vi "(SubVI)Waveform Editor_Import Manager_TextFile.vi"(6 "WF List_Sampling Rate":u32, 7 "New?":bool=TRUE, 8 "error in (no error)":errorcluster caption="에러 입력(에러 없음)", 10 "File Path":path=path "C:/Users/Oh Dae Woong/Desktop/test 221228.txt", 11 "Text File.lvclass":refnum<class "Text File.lvclass">) -> (0 "error out":errorcluster caption="에러 출력", 2 "Apply?":bool, 3 "Text File 출력":refnum<class "Text File.lvclass">)   [LabVIEW 2020]
uses:
  Libraries/Waveform Obj Class/Text File/Text File.lvclass
  Libraries/Waveform Obj Class/Waveform Obj/Waveform Obj.lvclass
  Libraries/Haptic IC Class/Haptic IC/Controls/(Ctrl)IC Type.ctl
  <vilib>/Utility/miscctls.llb/LVPointTypeDef.ctl
  Libraries/Waveform Obj Class/Waveform Obj/Waveform Obj.lvclass/Waveform Obj.ctl
  Libraries/Waveform Obj Class/Text File/Text File.lvclass/Text File.ctl
  Libraries/Waveform Obj Class/PWL_DW7802/PWL_DW7802.lvclass
  Libraries/Waveform Obj Class/PWL/PWL.lvclass/PWL.ctl
  Libraries/Waveform Obj Class/Waveform Gen/Waveform Gen.lvclass/Waveform Gen.ctl
  Libraries/Waveform Obj Class/Waveform Obj/Accessors/Read name.vi
  Libraries/Waveform Obj Class/Text File/Accessors/Read Text_Format.vi
  Libraries/Waveform Obj Class/Text File/Accessors/Read Text_Data.vi
  Libraries/Waveform Obj Class/Text File/Accessors/Read voltage idx.vi
  Libraries/Waveform Obj Class/Waveform Obj/Accessors/Read wait.vi
  Libraries/Waveform Obj Class/Waveform Obj/Accessors/Write sampling rate.vi
  Libraries/Waveform Obj Class/Text File/Accessors/Read Text_Sampling Rate.vi
  Libraries/Waveform Obj Class/Text File/Accessors/Read Text_ic type.vi
  Libraries/Waveform Obj Class/Waveform Obj/Accessors/Read play mode.vi
  Libraries/Waveform Obj Class/Text File/Accessors/Read Data.vi
  Libraries/Waveform Obj Class/Waveform Obj/Accessors/Write name.vi
  Libraries/Waveform Obj Class/PWL/Accessors/Write waveform type.vi
  Libraries/Waveform Obj Class/Waveform Gen/Accessors/Write repeat type.vi
  Libraries/Waveform Obj Class/Waveform Gen/Accessors/Write scale.vi
  Libraries/Waveform Obj Class/Waveform Gen/Accessors/Write frequency.vi
  Libraries/Waveform Obj Class/Waveform Gen/Accessors/Write cycle.vi
  Libraries/Waveform Obj Class/Waveform Obj/Accessors/Write play mode.vi
  Libraries/Waveform Obj Class/Waveform Obj/Accessors/Write voltage range.vi
  Libraries/Waveform Obj Class/PWL/Accessors/Write previous pwl scale.vi
  Libraries/Waveform Obj Class/Text File/Accessors/Read Text_File_PWL.vi
  Libraries/Waveform Obj Class/Waveform Obj/Accessors/Read sampling rate.vi
  Libraries/Waveform Obj Class/Text File/Accessors/Write voltage idx.vi
  Libraries/Waveform Obj Class/Waveform Obj/Accessors/Write wait.vi
  Libraries/Waveform Obj Class/Text File/Accessors/Read Error_.vi
  Libraries/Waveform Obj Class/Text File/Accessors/Read Memory Set.vi
  Variables/(Var)System Variables.vi
  <vilib>/Utility/file.llb/Write Delimited Spreadsheet (string).vi
  Libraries/Haptic IC Class/Haptic IC/Haptic IC.lvclass
panel:
  out "WAV_Sampling Rate":u32 caption="Sampling Rate" format="%#pHz"
  in  "Voltage Range":dbl(ring) caption="VD Clamp" items=["0.00V"=0.0, "0.04V"=0.04, "0.08V"=0.08, "0.12V"=0.12, "0.16V"=0.16, "0.20V"=0.2, "0.24V"=0.24, "0.28V"=0.28, "0.32V"=0.32, "0.36V"=0.36, "0.40V"=0.4, "0.44V"=0.44, "0.48V"=0.48, "0.52V"=0.52, "0.56V"=0.56, "0.60V"=0.6, "0.64V"=0.64, "0.68V"=0.68, "0.72V"=0.72, "0.76V"=0.76, "0.80V"=0.8, "0.84V"=0.84, "0.88V"=0.88, "0.92V"=0.92, "0.96V"=0.96, "1.00V"=1.0, "1.04V"=1.04, "1.08V"=1.08, "1.12V"=1.12, "1.16V"=1.16, "1.20V"=1.2, "1.24V"=1.24, "1.28V"=1.28, "1.32V"=1.32, "1.36V"=1.36, "1.40V"=1.4, "1.44V"=1.44, "1.48V"=1.48, "1.52V"=1.52, "1.56V"=1.56, "1.60V"=1.6, "1.64V"=1.64, "1.68V"=1.68, "1.72V"=1.72, "1.76V"=1.76, "1.80V"=1.8, "1.84V"=1.84, "1.88V"=1.88, "1.92V"=1.92, "1.96V"=1.96, "2.00V"=2.0, "2.04V"=2.04, "2.08V"=2.08, "2.12V"=2.12, "2.16V"=2.16, "2.20V"=2.2, "2.24V"=2.24, "2.28V"=2.28, "2.32V"=2.32, "2.36V"=2.36, "2.40V"=2.4, "2.44V"=2.44, "2.48V"=2.48, "2.52V"=2.52, "2.56V"=2.56, "2.60V"=2.6, "2.64V"=2.64, "2.68V"=2.68, "2.72V"=2.72, "2.76V"=2.76, "2.80V"=2.8, "2.84V"=2.84, "2.88V"=2.88, "2.92V"=2.92, "2.96V"=2.96, "3.00V"=3.0, "3.04V"=3.04, "3.08V"=3.08, "3.12V"=3.12, "3.16V"=3.16, "3.20V"=3.2, "3.24V"=3.24, "3.28V"=3.28, "3.32V"=3.32, "3.36V"=3.36, "3.40V"=3.4, "3.44V"=3.44, "3.48V"=3.48, "3.52V"=3.52, "3.56V"=3.56, "3.60V"=3.6, "3.64V"=3.64, "3.68V"=3.68, "3.72V"=3.72, "3.76V"=3.76, "3.80V"=3.8, "3.84V"=3.84, "3.88V"=3.88, "3.92V"=3.92, "3.96V"=3.96, "4.00V"=4.0, "4.04V"=4.04, "4.08V"=4.08, "4.12V"=4.12, "4.16V"=4.16, "4.20V"=4.2, "4.24V"=4.24, "4.28V"=4.28, "4.32V"=4.32, "4.36V"=4.36, "4.40V"=4.4, "4.44V"=4.44, "4.48V"=4.48, "4.52V"=4.52, "4.56V"=4.56, "4.60V"=4.6, "4.64V"=4.64, "4.68V"=4.68, "4.72V"=4.72, "4.76V"=4.76, "4.80V"=4.8, "4.84V"=4.84, "4.88V"=4.88, "4.92V"=4.92, "4.96V"=4.96, "5.00V"=5.0, "5.04V"=5.04, "5.08V"=5.08, "5.12V"=5.12, "5.16V"=5.16, "5.20V"=5.2, "5.24V"=5.24, "5.28V"=5.28, "5.32V"=5.32, "5.36V"=5.36, "5.40V"=5.4, "5.44V"=5.44, "5.48V"=5.48, "5.52V"=5.52, "5.56V"=5.56, "5.60V"=5.6, "5.64V"=5.64, "5.68V"=5.68, "5.72V"=5.72, "5.76V"=5.76, "5.80V"=5.8, "5.84V"=5.84, "5.88V"=5.88, "5.92V"=5.92, "5.96V"=5.96, "6.00V"=6.0, "6.04V"=6.04, "6.08V"=6.08, "6.12V"=6.12, "6.16V"=6.16, "6.20V"=6.2, "6.24V"=6.24, "6.28V"=6.28, "6.32V"=6.32, "6.36V"=6.36, "6.40V"=6.4, "6.44V"=6.44, "6.48V"=6.48, "6.52V"=6.52, "6.56V"=6.56, "6.60V"=6.6, "6.64V"=6.64, "6.68V"=6.68, "6.72V"=6.72, "6.76V"=6.76, "6.80V"=6.8, "6.84V"=6.84, "6.88V"=6.88, "6.92V"=6.92, "6.96V"=6.96, "7.00V"=7.0, "7.04V"=7.04, "7.08V"=7.08, "7.12V"=7.12, "7.16V"=7.16, "7.20V"=7.2, "7.24V"=7.24, "7.28V"=7.28, "7.32V"=7.32, "7.36V"=7.36, "7.40V"=7.4, "7.44V"=7.44, "7.48V"=7.48, "7.52V"=7.52, "7.56V"=7.56, "7.60V"=7.6, "7.64V"=7.64, "7.68V"=7.68, "7.72V"=7.72, "7.76V"=7.76, "7.80V"=7.8, "7.84V"=7.84, "7.88V"=7.88, "7.92V"=7.92, "7.96V"=7.96, "8.00V"=8.0, "8.04V"=8.04, "8.08V"=8.08, "8.12V"=8.12, "8.16V"=8.16, "8.20V"=8.2, "8.24V"=8.24, "8.28V"=8.28, "8.32V"=8.32, "8.36V"=8.36, "8.40V"=8.4, "8.44V"=8.44, "8.48V"=8.48, "8.52V"=8.52, "8.56V"=8.56, "8.60V"=8.6, "8.64V"=8.64, "8.68V"=8.68, "8.72V"=8.72, "8.76V"=8.76, "8.80V"=8.8, "8.84V"=8.84, "8.88V"=8.88, "8.92V"=8.92, "8.96V"=8.96, "9.00V"=9.0, "9.04V"=9.04, "9.08V"=9.08, "9.12V"=9.12, "9.16V"=9.16, "9.20V"=9.2, "9.24V"=9.24, "9.28V"=9.28, "9.32V"=9.32, "9.36V"=9.36, "9.40V"=9.4, "9.44V"=9.44, "9.48V"=9.48, "9.52V"=9.52, "9.56V"=9.56, "9.60V"=9.6, "9.64V"=9.64, "9.68V"=9.68, "9.72V"=9.72, "9.76V"=9.76, "9.80V"=9.8, "9.84V"=9.84, "9.88V"=9.88, "9.92V"=9.92, "9.96V"=9.96, "10.00V"=10.0, "10.04V"=10.04, "10.08V"=10.08, "10.12V"=10.12, "10.16V"=10.16, "10.20V"=10.2]
  in  "WF Gen":refnum<class "Waveform Obj.lvclass">
  in  "IC TYPE TAB":enum32{"DW7914", "DW7802"}(tab)
  in  "Wait":u8(ring) items=["0us", "166us", "332us", "498us", "664us", "830us", "996us", "1162us", "1328us", "1494us", "1660us", "1826us", "1992us", "2158us", "2324us", "2490us"]
  out "WF Seq_Play Mode":u8(ring) caption="Play Mode" items=["Direct Playback Mode", "Synthesis Playback Mode"]
  in  "play mode tab":enum32{"DW7914", "DW7802"}(tab)
  out "TXT_EOL+Delimiter":bool=TRUE
  out "TXT_End of LIne":enum16{"EOL (\\r\\n)", "LF (\\n)"}(ring) caption="End of Line"
  out "TXT_Number per Line":i32=1 caption="Number per Line" min=1 max=100
  out "TXT_Delimiter":string(combo)="\r\n" caption="Delimiter"
  out "TXT_Prefix":bool=TRUE
  out "TXT_Radix":enum16{"BIN", "DEC", "HEX"}(ring)=enum."HEX" caption="Radix"
  out "WF Seq_PWL_DW7802 3":T1(array[cluster])=[{"Shape"=0, "Ramp"=0, "Amplitude"=1.0, "Frequency"=100.0, "Cycle"=1.0}] {"Frequency" min=40.0 max=300.0 step=1.0; "Cycle" items=["0.5"=0.5, "1"=1.0, "1.5"=1.5, "2"=2.0, "2.5"=2.5, "3"=3.0, "3.5"=3.5, "4"=4.0, "4.5"=4.5, "5"=5.0, "5.5"=5.5, "6"=6.0, "6.5"=6.5, "7"=7.0, "7.5"=7.5, "8"=8.0, "8.5"=8.5, "9"=9.0, "9.5"=9.5, "10"=10.0, "10.5"=10.5, "11"=11.0, "11.5"=11.5, "12"=12.0, "12.5"=12.5, "13"=13.0, "13.5"=13.5, "14"=14.0, "14.5"=14.5, "15"=15.0, "15.5"=15.5, "16"=16.0, "16.5"=16.5, "17"=17.0, "17.5"=17.5, "18"=18.0, "18.5"=18.5, "19"=19.0, "19.5"=19.5, "20"=20.0, "20.5"=20.5, "21"=21.0, "21.5"=21.5, "22"=22.0, "22.5"=22.5, "23"=23.0, "23.5"=23.5, "24"=24.0, "24.5"=24.5, "25"=25.0, "25.5"=25.5, "26"=26.0, "26.5"=26.5, "27"=27.0, "27.5"=27.5, "28"=28.0, "28.5"=28.5, "29"=29.0, "29.5"=29.5, "30"=30.0, "30.5"=30.5, "31"=31.0, "31.5"=31.5, "32"=32.0, "32.5"=32.5, "33"=33.0, "33.5"=33.5, "34"=34.0, "34.5"=34.5, "35"=35.0, "35.5"=35.5, "36"=36.0, "36.5"=36.5, "37"=37.0, "37.5"=37.5, "38"=38.0, "38.5"=38.5, "39"=39.0, "39.5"=39.5, "40"=40.0, "40.5"=40.5, "41"=41.0, "41.5"=41.5, "42"=42.0, "42.5"=42.5, "43"=43.0, "43.5"=43.5, "44"=44.0, "44.5"=44.5, "45"=45.0, "45.5"=45.5, "46"=46.0, "46.5"=46.5, "47"=47.0, "47.5"=47.5, "48"=48.0, "48.5"=48.5, "49"=49.0, "49.5"=49.5, "50"=50.0, "50.5"=50.5, "51"=51.0, "51.5"=51.5, "52"=52.0, "52.5"=52.5, "53"=53.0, "53.5"=53.5, "54"=54.0, "54.5"=54.5, "55"=55.0, "55.5"=55.5, "56"=56.0, "56.5"=56.5, "57"=57.0, "57.5"=57.5, "58"=58.0, "58.5"=58.5, "59"=59.0, "59.5"=59.5, "60"=60.0, "60.5"=60.5, "61"=61.0, "61.5"=61.5, "62"=62.0, "62.5"=62.5, "63"=63.0, "63.5"=63.5, "64"=64.0, "64.5"=64.5, "65"=65.0, "65.5"=65.5, "66"=66.0, "66.5"=66.5, "67"=67.0, "67.5"=67.5, "68"=68.0, "68.5"=68.5, "69"=69.0, "69.5"=69.5, "70"=70.0, "70.5"=70.5, "71"=71.0, "71.5"=71.5, "72"=72.0, "72.5"=72.5, "73"=73.0, "73.5"=73.5, "74"=74.0, "74.5"=74.5, "75"=75.0, "75.5"=75.5, "76"=76.0, "76.5"=76.5, "77"=77.0, "77.5"=77.5, "78"=78.0, "78.5"=78.5, "79"=79.0, "79.5"=79.5, "80"=80.0, "80.5"=80.5, "81"=81.0, "81.5"=81.5, "82"=82.0, "82.5"=82.5, "83"=83.0, "83.5"=83.5, "84"=84.0, "84.5"=84.5, "85"=85.0, "85.5"=85.5, "86"=86.0, "86.5"=86.5, "87"=87.0, "87.5"=87.5, "88"=88.0, "88.5"=88.5, "89"=89.0, "89.5"=89.5, "90"=90.0, "90.5"=90.5, "91"=91.0, "91.5"=91.5, "92"=92.0, "92.5"=92.5, "93"=93.0, "93.5"=93.5, "94"=94.0, "94.5"=94.5, "95"=95.0, "95.5"=95.5, "96"=96.0, "96.5"=96.5, "97"=97.0, "97.5"=97.5, "98"=98.0, "98.5"=98.5, "99"=99.0, "99.5"=99.5, "100"=100.0, "100.5"=100.5, "101"=101.0, "101.5"=101.5, "102"=102.0, "102.5"=102.5, "103"=103.0, "103.5"=103.5, "104"=104.0, "104.5"=104.5, "105"=105.0, "105.5"=105.5, "106"=106.0, "106.5"=106.5, "107"=107.0, "107.5"=107.5, "108"=108.0, "108.5"=108.5, "109"=109.0, "109.5"=109.5, "110"=110.0, "110.5"=110.5, "111"=111.0, "111.5"=111.5, "112"=112.0, "112.5"=112.5, "113"=113.0, "113.5"=113.5, "114"=114.0, "114.5"=114.5, "115"=115.0, "115.5"=115.5, "116"=116.0, "116.5"=116.5, "117"=117.0, "117.5"=117.5, "118"=118.0, "118.5"=118.5, "119"=119.0, "119.5"=119.5, "120"=120.0, "120.5"=120.5, "121"=121.0, "121.5"=121.5, "122"=122.0, "122.5"=122.5, "123"=123.0, "123.5"=123.5, "124"=124.0, "124.5"=124.5, "125"=125.0, "125.5"=125.5, "126"=126.0, "126.5"=126.5, "127"=127.0, "127.5"=127.5]; "Amplitude" items=["0"=0.0, "10"=0.1, "20"=0.2, "30"=0.3, "40"=0.4, "50"=0.5, "60"=0.6, "70"=0.7, "80"=0.8, "90"=0.9, "100"=1.0]; "Ramp" items=["Step"=0, "Ramp (Lin.)"=2, "Ramp (Exp.)"=3]; "Shape" items=["Sine", "Square"]}
  out "WF Seq_PWL Listbox":i32[](listbox)
  out "Input WF List_Sampling Rate":u32
  out "TXT_Preview":string caption="Preview"
  in  "Apply":bool
  out "Graph":waveform(dbl)(graph)
  # "Import Manager"
  # "Data Format"
  # "Preview"
  # "Data"
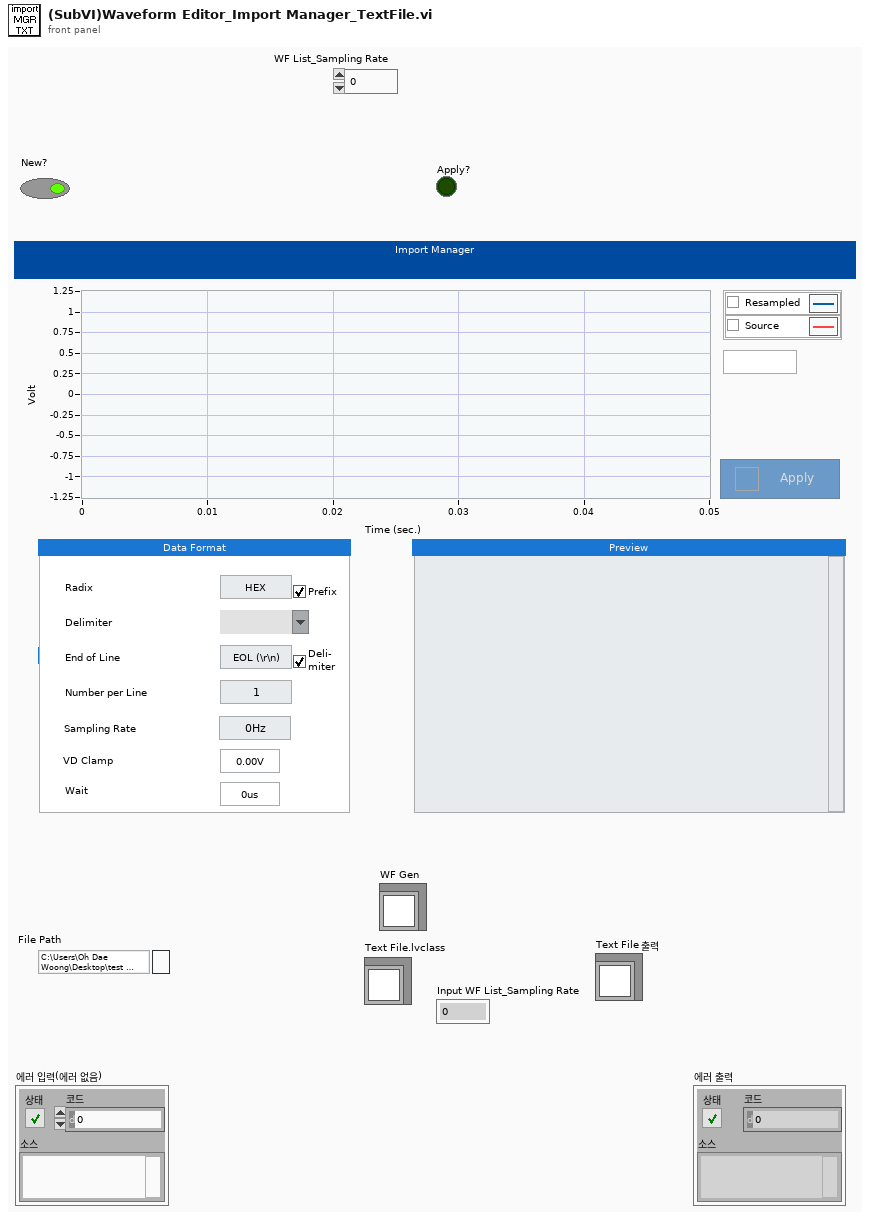
[diagram p1: front panel]
types:
  T1 = cluster{"Shape":u16, "Ramp":u16, "Amplitude":dbl, "Frequency":dbl, "Cycle":dbl}[]
  T2 = typedef "Haptic IC.lvclass/(Ctrl)IC Type.ctl" = enum8{"DW7800", "DW7802", "DW7912", "DW7914"}
  T3 = enum8{"Enabled", "Disabled", "Disabled and Grayed Out"}
  T4 = typedef "LVPointTypeDef.ctl" = cluster{"Horizontal":i16, "Vertical":i16}
  T5 = typedef "LVStringsAndValuesArrayTypeDef_DBL.ctl" = cluster{"String":string, "Value":dbl}[]
  T6 = typedef "LVStringsAndValuesArrayTypeDef_U8.ctl" = cluster{"String":string, "Value":u8}[]
  T7 = cluster{"TXT_Radix":enum16{"BIN", "DEC", "HEX"}, "TXT_Prefix":bool, "TXT_Delimiter":string, "TXT_End of LIne":enum16{"EOL (\\r\\n)", "LF (\\n)"}, "TXT_EOL+Delimiter":bool, "TXT_Number per Line":i32}
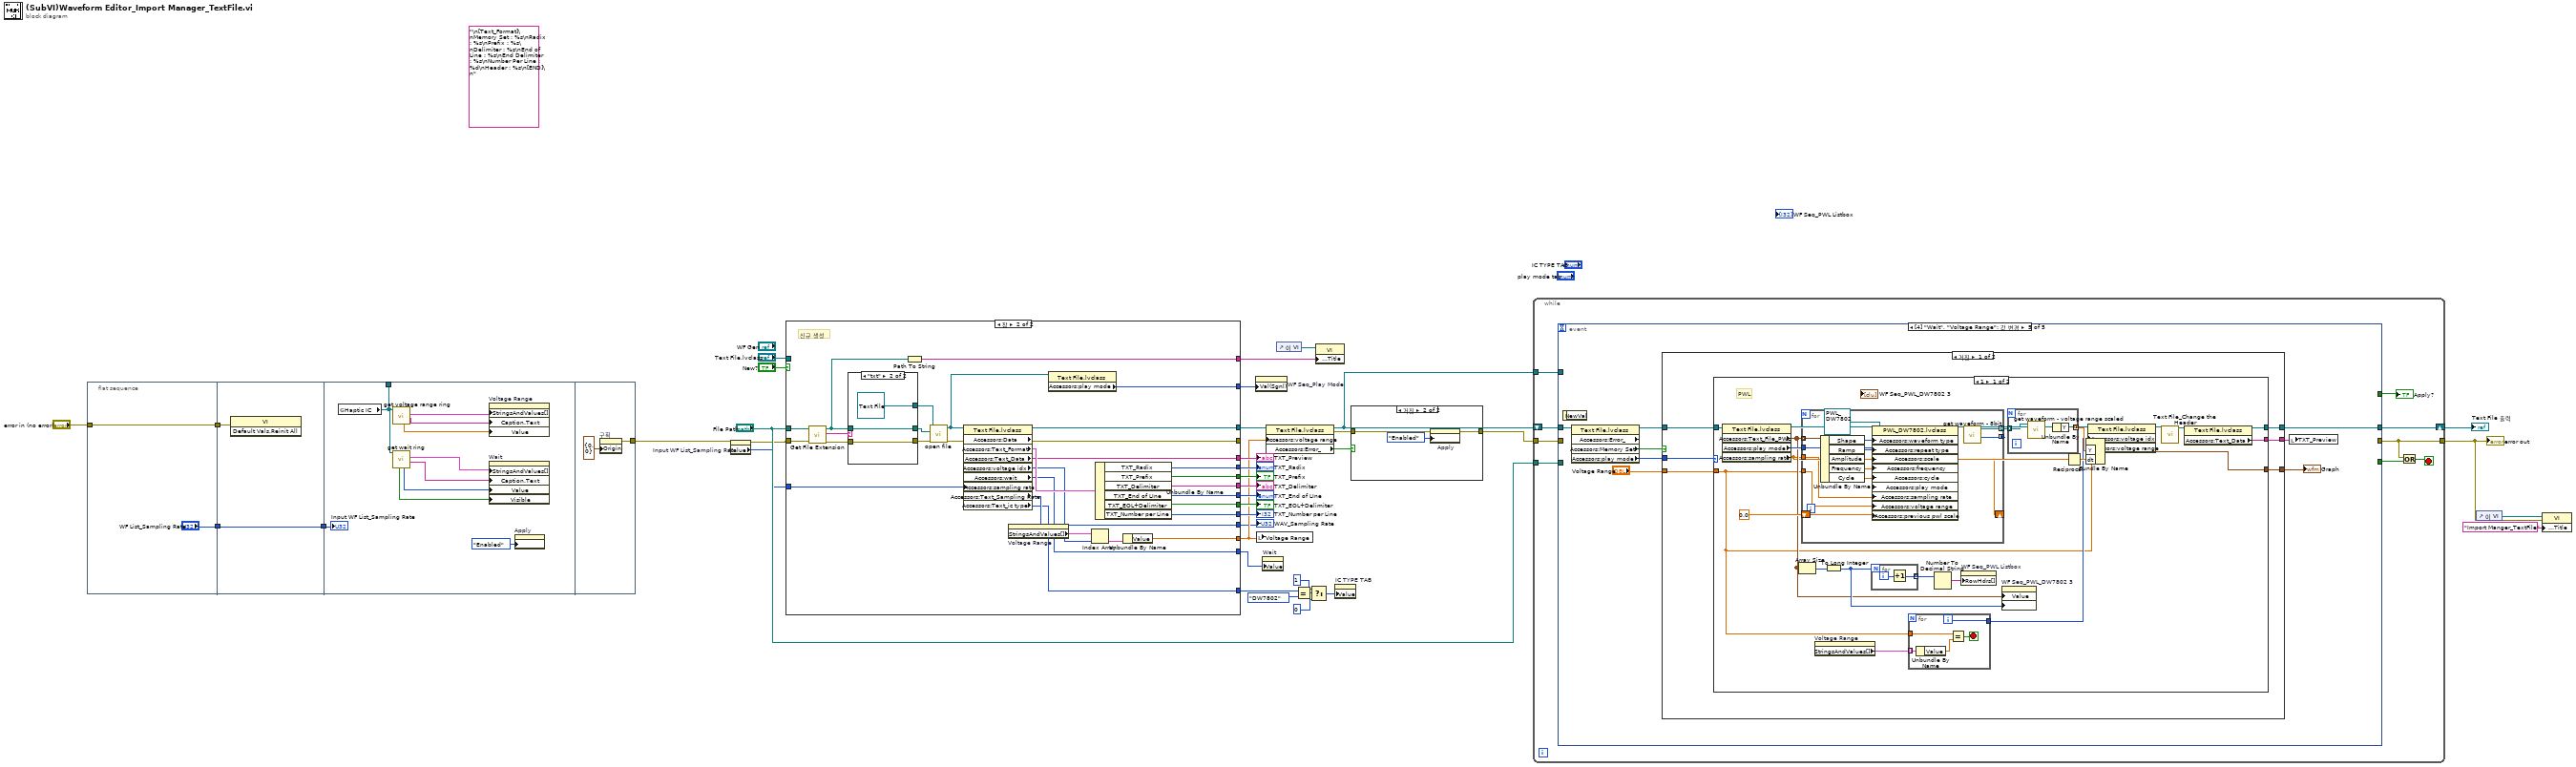
[diagram p0: block diagram]
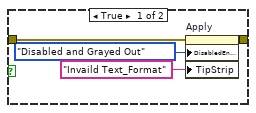
[diagram p2: hidden frame]
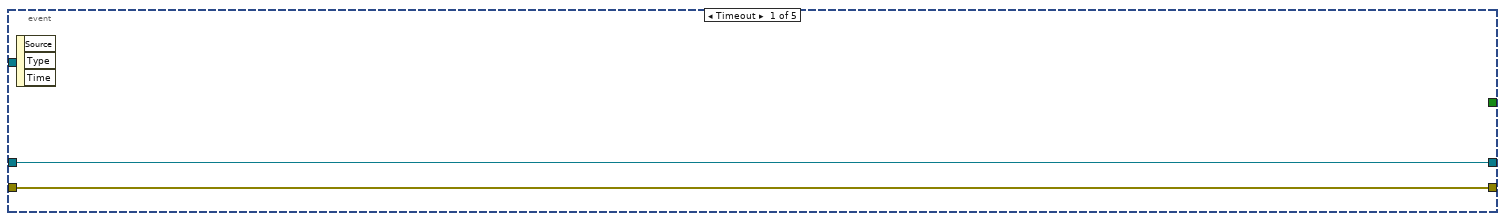
[diagram p3: hidden frame]
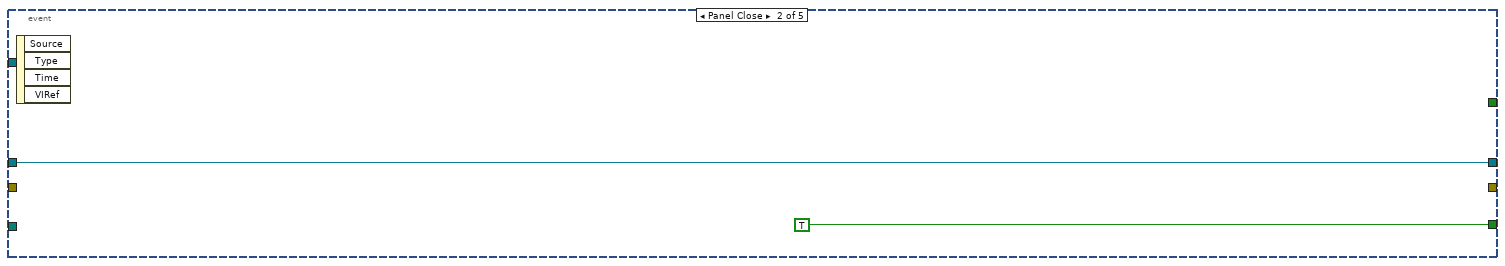
[diagram p4: hidden frame]
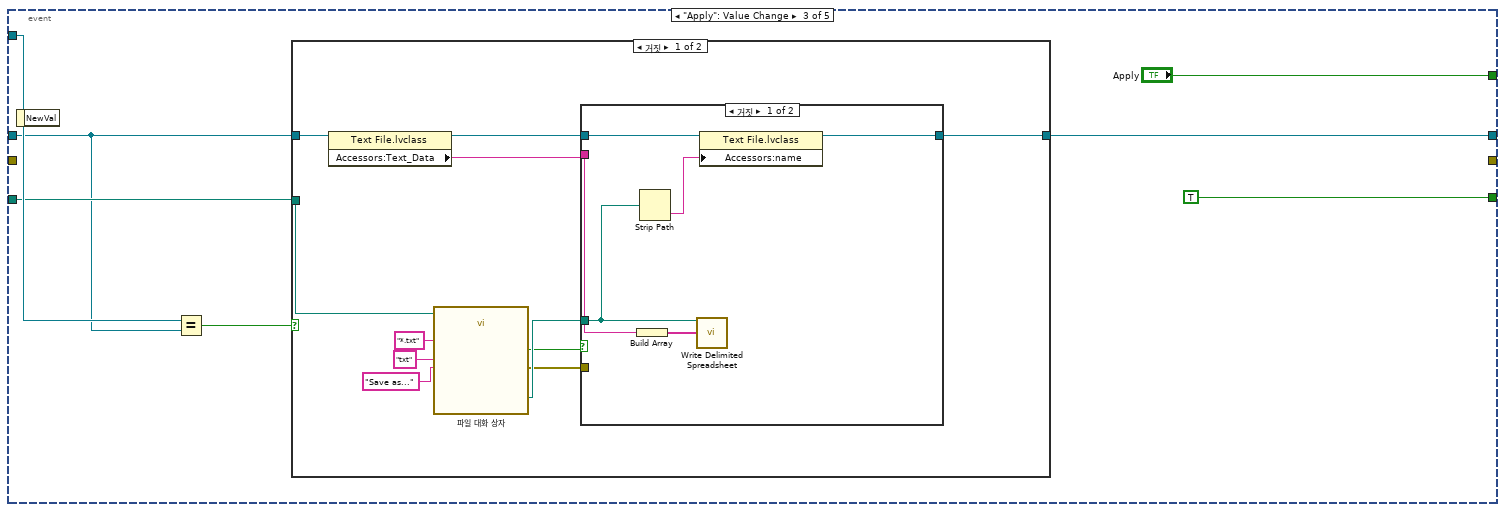
[diagram p5: hidden frame]
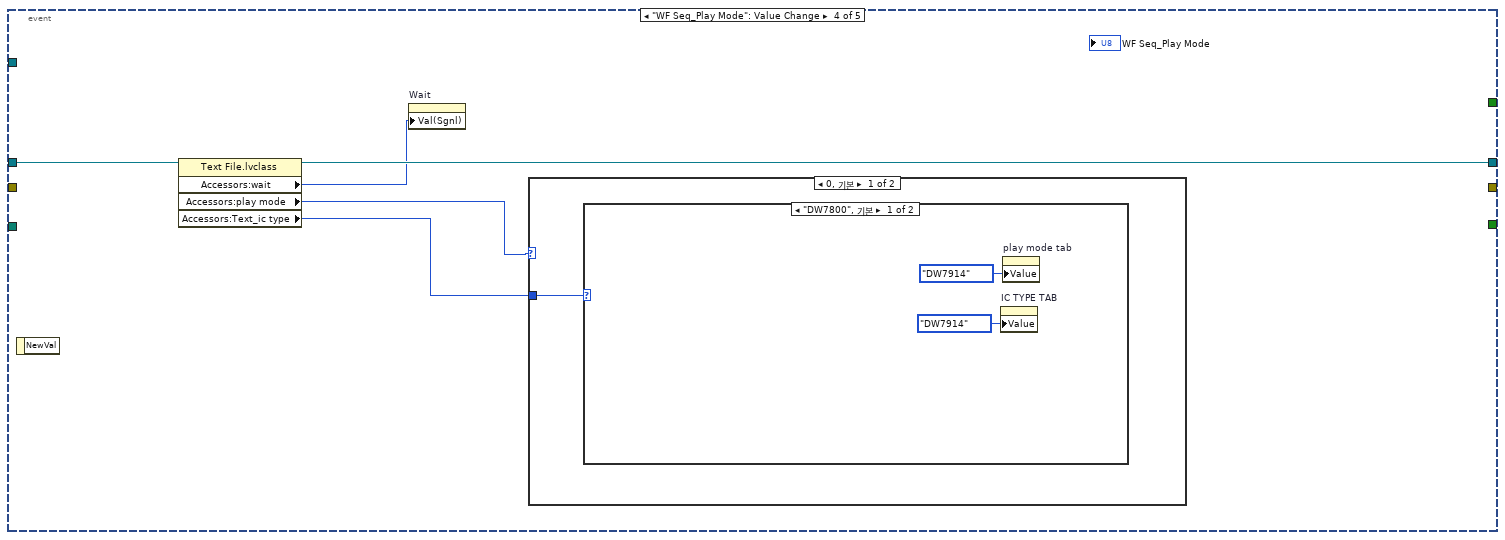
[diagram p8: hidden frame]
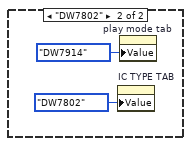
[diagram p9: hidden frame]
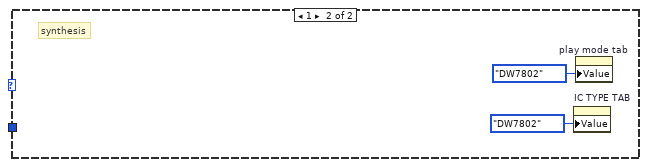
[diagram p10: hidden frame]
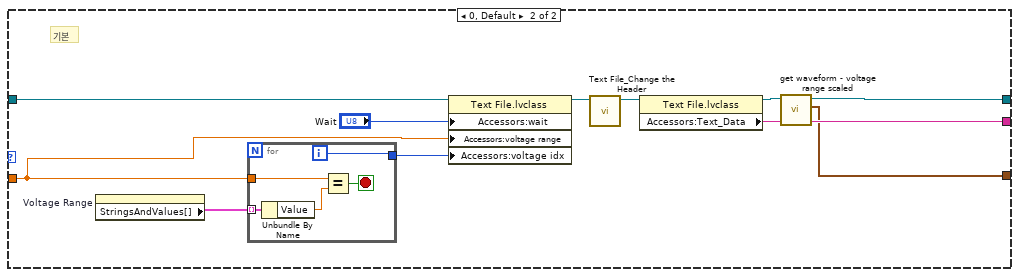
[diagram p11: hidden frame]
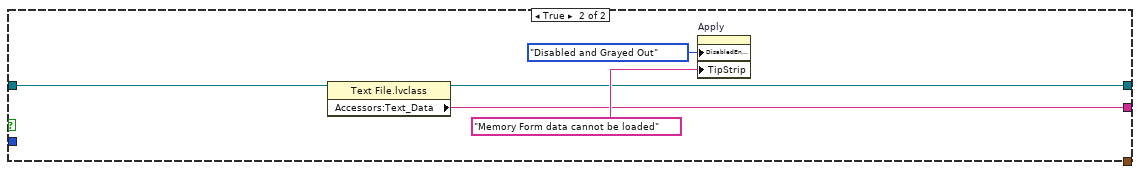
[diagram p12: hidden frame]
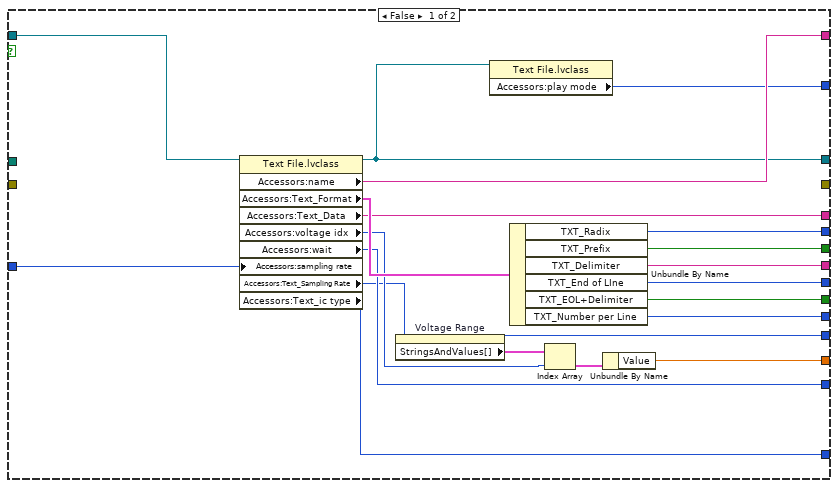
[diagram p13: hidden frame]
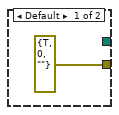
[diagram p14: hidden frame]
diagram:
  (unwired) "\n[Text_Format]\nMemory Set : %s\nRadix : %s\nPrefix : %s\nDelimiter : %s\nEnd of Line : %s\nEnd Delimiter : %s\nNumber Per Line : %d\nHeader : %s\n[END]\n" ("포맷 문자열")
  n1 = flat-sequence {
    tunnel: "error in (no error)" -> [w40]
    tunnel: [w40] -> w22
    tunnel: ["WF List_Sampling Rate"] -> w20
    tunnel: w22 -> [w42]
    tunnel: [w41] -> w21
    tunnel: w20 -> [w41]
    tunnel: w21 -> [w45]
    tunnel: [w43] -> _
    tunnel: [w53] -> w18
    frame #0 {
    }
    frame #1 {
      n2 = invoke class="VI" method="Default Vals.Reinit All"(error in=w42) -> ()  [unwired: 2 in, 3 out]
    }
    frame #2 {
      n3 = global read "(Var)System Variables.vi" "Haptic IC"() -> (w43:refnum<class "Haptic IC.lvclass">)
      n4 = call-dynamic "get voltage range ring.vi"("Haptic IC 입력"=w43) -> ("caption"=w47:string, "strings & values"=w46:T5, "read value"=w48:dbl)  [unwired: 6 in, 2 out]
      n5 = call-dynamic "get wait ring.vi"("Haptic IC 입력"=w43) -> ("caption"=w50:string, "strings & values"=w49:T6, "default value"=w51:u8, "using"=w52:bool)  [unwired: 5 in, 2 out]
      n6 = property on="Voltage Range" class="Ring (엄격한)"("StringsAndValues[]"=w46, "Caption.Text"=w47, "Value"=w48) -> ()  [unwired: 2 in, 2 out]
      n7 = property on="Wait" class="Ring (엄격한)"("StringsAndValues[]"=w49, "Caption.Text"=w50, "Value"=w51, "Visible"=w52) -> ()  [unwired: 2 in, 2 out]
      n8 = property on="Apply" class="Bool"("DisabledEnum"=T3."Enabled" ("비활성화")) -> ()  [unwired: 2 in, 2 out]
      "Input WF List_Sampling Rate" <- w45
    }
    frame #3 {
      n9 = property on="구획" class="Pane"("Origin"=T4 {"Horizontal"=0, "Vertical"=0} ("원점")) -> (error out=w53:errorcluster)  [unwired: 2 in, 1 out]
    }
  }
  n10 = property on="Input WF List_Sampling Rate" class="DigNum (엄격한)"(error in=w18) -> (error out=w17:errorcluster, "Value"=w16:u32)  [unwired: 1 in, 1 out]
  n11 = case shown="참" "New?" {
    tunnel: w17 -> [_ w103]
    tunnel: "Text File.lvclass" -> [w73 _]
    tunnel: "File Path" -> [_ w102]
    tunnel: [_ w95] -> _
    tunnel: [w56 w87] -> w26
    tunnel: [w72 w94] -> w35
    tunnel: [w67 w93] -> w34
    tunnel: [w69 w92] -> w33
    tunnel: [w68 w91] -> w32
    tunnel: [w70 w90] -> w31
    tunnel: [w71 w89] -> w30
    tunnel: [w66 w88] -> w29
    tunnel: [w62 w83] -> w28
    tunnel: [w61 w82] -> w27
    tunnel: [w60 w81] -> w19
    tunnel: w16 -> [w59 w80]
    tunnel: [w58 w78] -> w15
    tunnel: [w57 w77] -> w4
    tunnel: [w55 w75] -> w5
    frame False {
      n12 = property class="Text File.lvclass"(reference=w73, "Accessors:sampling rate"=w59) -> (reference out=w56:refnum<class "Text File.lvclass">, "Accessors:name"=w58:string, "Accessors:Text_Format"=w74:T7, "Accessors:Text_Data"=w72:string, "Accessors:voltage idx"=w63:i32, "Accessors:wait"=w61:u8, "Accessors:Text_Sampling Rate"=w60:i32, "Accessors:Text_ic type"=w57:T2)  [unwired: 1 in, 1 out]
      n13 = property on="Voltage Range" class="Ring (엄격한)"() -> ("StringsAndValues[]"=w65:T5)  [unwired: 2 in, 2 out]
      n14 = property class="Text File.lvclass"(reference=w56) -> ("Accessors:play mode"=w55:u8)  [unwired: 1 in, 2 out]
      n15 = Unbundle By Name(w74) -> ("TXT_Radix"=w66:enum16{"BIN", "DEC", "HEX"}, "TXT_Prefix"=w71:bool, "TXT_Delimiter"=w70:string, "TXT_End of LIne"=w69:enum16{"EOL (\\r\\n)", "LF (\\n)"}, "TXT_EOL+Delimiter"=w68:bool, "TXT_Number per Line"=w67:i32)
      n16 = Index Array(array=w65, index=w63) -> (element=w64:cluster{"String":string, "Value":dbl})
      n17 = Unbundle By Name(w64) -> ("Value"=w62:dbl)
    }
    frame True {
      # "신규 생성"
      n18 = call <vilib>:"Get File Extension.vi"("error in (no error)"=w103, "file"=w102) -> ("error out"=w101:errorcluster, "lowercase file extension"=w100:string, "dup file"=w79:path)  [unwired: 5 in, 2 out]
      n19 = case shown="\"txt\"" w100 {
        tunnel: w101 -> [_ w107]
        tunnel: [errorcluster {"status"=TRUE, "code"=0, "source"=""} ("error out") w107] -> w98
        tunnel: [_ refnum<class "Text File.lvclass"> refnum ("Text File.lvclass")] -> w99
        tunnel: w79 -> [_ w106]
        tunnel: [_ w106] -> w97
        frame Default {
        }
        frame "txt" {
        }
      }
      n20 = Path To String(path=w79) -> (string=w78:string)
      n21 = call-dynamic "open file.vi"("error in (no error)"=w98, "file path"=w97, "Text File 입력"=w99) -> ("error out"=w95:errorcluster, "Text File 출력"=w76:refnum<class "Text File.lvclass">)  [unwired: 7 in]
      n22 = property class="Text File.lvclass" props=["Accessors:Data", "Accessors:Text_Format", "Accessors:Text_Data", "Accessors:voltage idx", "Accessors:wait", "Accessors:sampling rate", "Accessors:Text_Sampling Rate", "Accessors:Text_ic type"](reference=w76, "Accessors:sampling rate"=w80) -> (reference out=w87:refnum<class "Text File.lvclass">, "Accessors:Text_Format"=w96:T7, "Accessors:Text_Data"=w94:string, "Accessors:voltage idx"=w85:i32, "Accessors:wait"=w82:u8, "Accessors:Text_Sampling Rate"=w81:i32, "Accessors:Text_ic type"=w77:T2)  [unwired: 1 in, 2 out]
      n23 = property on="Voltage Range" class="Ring (엄격한)"() -> ("StringsAndValues[]"=w86:T5)  [unwired: 2 in, 2 out]
      n24 = property class="Text File.lvclass"(reference=w76) -> ("Accessors:play mode"=w75:u8)  [unwired: 1 in, 2 out]
      n25 = Index Array(array=w86, index=w85) -> (element=w84:cluster{"String":string, "Value":dbl})
      n26 = Unbundle By Name(w96) -> ("TXT_Radix"=w88:enum16{"BIN", "DEC", "HEX"}, "TXT_Prefix"=w89:bool, "TXT_Delimiter"=w90:string, "TXT_End of LIne"=w92:enum16{"EOL (\\r\\n)", "LF (\\n)"}, "TXT_EOL+Delimiter"=w91:bool, "TXT_Number per Line"=w93:i32)
      n27 = Unbundle By Name(w84) -> ("Value"=w83:dbl)
    }
  }
  "TXT_Radix" <- w29
  "TXT_Prefix" <- w30
  "TXT_Delimiter" <- w31
  "TXT_EOL+Delimiter" <- w32
  "TXT_End of LIne" <- w33
  "TXT_Number per Line" <- w34
  "TXT_Preview" <- w35
  "WAV_Sampling Rate" <- w19
  n28 = property on="WF Seq_Play Mode" class="Ring (엄격한)"("Val(Sgnl)"=w5) -> ()  [unwired: 2 in, 2 out]
  n29 = local write "Voltage Range"(w28) -> ()
  n30 = property on="Wait" class="Ring (엄격한)"("Value"=w27) -> ()  [unwired: 2 in, 2 out]
  n31 = property class="Text File.lvclass"(reference=w26, "Accessors:voltage range"=w28) -> (reference out=w24:refnum<class "Text File.lvclass">, error out=w3:errorcluster, "Accessors:Error_"=w1:bool)  [unwired: 1 in]
  n32 = control-ref of="이 VI"() -> (w14:refnum<vi>)
  n33 = Equal?(x=w4, y=(Ctrl)IC_Type."DW7802") -> (x = y?=w9:bool)
  n34 = Select(t=1, s=w9, f=0) -> (s? t:f=w6:i32)
  n35 = property class="VI"(reference=w14, "Front Panel.Title"=w15) -> ()  [unwired: 1 in, 2 out]
  n36 = property on="IC TYPE TAB" class="TabCtl (엄격한)"("Value"=w6) -> ()  [unwired: 2 in, 2 out]
  n37 = case shown="거짓" w1 {
    tunnel: w3 -> [w109 w113]
    tunnel: [w108 w112] -> w2
    frame True {
      n38 = property on="Apply" class="Bool"(error in=w109, "DisabledEnum"=T3."Disabled and Grayed Out" ("비활성화"), "TipStrip"="Invaild Text_Format" ("설명")) -> (error out=w108:errorcluster)  [unwired: 1 in, 1 out]
    }
    frame False {
      n39 = property on="Apply" class="Bool"(error in=w113, "DisabledEnum"=T3."Enabled" ("비활성화")) -> (error out=w112:errorcluster)  [unwired: 1 in, 1 out]
    }
  }
  n40 = while {
    tunnel: w2 -> [w123]
    tunnel: [w121] -> w11
    tunnel: w24 -> [w117]
    tunnel: "File Path" -> [w116]
    shift-right: [w115] -> w23
    shift-left: w24 -> [w122]
    stop <- w120 stop-if-true
    n41 = event shown="[4] \"Wait\", \"Voltage Range\": 값 변경" {
      selector: _ -> [_ _ _ _ _]
      dyn-events: _ -> [_ _ _ _ _]
      timeout: _ -> [_ _ _ _ _]
      tunnel: w123 -> [w124 _ _ _ _]
      tunnel: w122 -> [w125 w126 w129 w158 w173]
      tunnel: [w124 _ _ _ _] -> w121
      tunnel: [_ TRUE TRUE _ _] -> w119
      tunnel: [_ _ "Apply" _ _] -> w118
      tunnel: w117 -> [_ _ w132 _ _]
      tunnel: w116 -> [_ _ w130 _ _]
      tunnel: [w125 w126 w128 w157 w171] -> w115
      event Timeout {
        n42 = event-data() -> ()  [unwired: 1 in, 3 out]
      }
      event Panel Close {
        n43 = event-data() -> ()  [unwired: 1 in, 4 out]
      }
      event "Apply": Value Change {
        n44 = event-data() -> ()  [unwired: 1 in, 1 out]
        n45 = Equal?(x=w132, y=w129) -> (x = y?=w131:bool)
        n46 = case shown="거짓" w131 {
          tunnel: w130 -> [w145 _]
          tunnel: w129 -> [w140 w153]
          tunnel: [w137 w153] -> w128
          frame False {
            n47 = property class="Text File.lvclass"(reference=w140) -> (reference out=w138:refnum<class "Text File.lvclass">, "Accessors:Text_Data"=w139:string)  [unwired: 1 in, 1 out]
            n48 = call "파일 대화 상자"("start path"=w145, "prompt"="Save as..." ("default name"), "pattern (all files)"="*.txt", "pattern label"="txt") -> ("selected path"=w142:path, "cancelled"=w141:bool, "error out"=w136:errorcluster)  [unwired: 8 in, 1 out]
            n49 = case shown="거짓" w141 {
              tunnel: w142 -> [w148 _]
              tunnel: w139 -> [w146 _]
              tunnel: w138 -> [w150 w152]
              tunnel: [w149 w152] -> w137
              tunnel: w136 -> [_ _]
              frame False {
                n50 = Build Array(w146) -> (w151:string[])
                n51 = Strip Path(path=w148) -> (name=w147:string)  [unwired: 1 out]
                n52 = call-poly <vilib>:"Write Delimited Spreadsheet.vi"("file path (dialog if empty)"=w148, "1D data"=w151) -> ()  [unwired: 12 in, 2 out]
                n53 = property class="Text File.lvclass"(reference=w150, "Accessors:name"=w147) -> (reference out=w149:refnum<class "Text File.lvclass">)  [unwired: 1 in, 1 out]
              }
              frame True {
              }
            }
          }
          frame True {
          }
        }
      }
      event "WF Seq_Play Mode": Value Change {
        n54 = event-data() -> ()  [unwired: 1 in, 1 out]
        n55 = property class="Text File.lvclass"(reference=w158) -> (reference out=w157:refnum<class "Text File.lvclass">, "Accessors:wait"=w156:u8, "Accessors:play mode"=w155:u8, "Accessors:Text_ic type"=w154:T2)  [unwired: 1 in, 1 out]
        n56 = property on="Wait" class="Ring (엄격한)"("Val(Sgnl)"=w156) -> ()  [unwired: 2 in, 2 out]
        n57 = case shown="0, 기본" w155 {
          tunnel: w154 -> [w159 _]
          frame 0, Default {
            n58 = case shown="\"DW7800\", 기본" w159 {
              frame "DW7800", Default {
                n59 = property on="IC TYPE TAB" class="TabCtl (엄격한)"("Value"=enum32{"DW7914", "DW7802"}."DW7914" ("IC TYPE TAB")) -> ()  [unwired: 2 in, 2 out]
                n60 = property on="play mode tab" class="TabCtl (엄격한)"("Value"=enum32{"DW7914", "DW7802"}."DW7914" ("play mode tab")) -> ()  [unwired: 2 in, 2 out]
              }
              frame "DW7802" {
                n61 = property on="IC TYPE TAB" class="TabCtl (엄격한)"("Value"=enum32{"DW7914", "DW7802"}."DW7802" ("IC TYPE TAB")) -> ()  [unwired: 2 in, 2 out]
                n62 = property on="play mode tab" class="TabCtl (엄격한)"("Value"=enum32{"DW7914", "DW7802"}."DW7914" ("play mode tab")) -> ()  [unwired: 2 in, 2 out]
              }
            }
          }
          frame 1 {
            # "synthesis"
            n63 = property on="IC TYPE TAB" class="TabCtl (엄격한)"("Value"=enum32{"DW7914", "DW7802"}."DW7802" ("IC TYPE TAB")) -> ()  [unwired: 2 in, 2 out]
            n64 = property on="play mode tab" class="TabCtl (엄격한)"("Value"=enum32{"DW7914", "DW7802"}."DW7802" ("play mode tab")) -> ()  [unwired: 2 in, 2 out]
          }
        }
      }
      event "Wait", "Voltage Range": Value Change {
        n65 = event-data() -> ()  [unwired: 1 in, 1 out]
        n66 = property class="Text File.lvclass" props=["Accessors:Error_", "Accessors:Memory Set", "Accessors:play mode"](reference=w173) -> (reference out=w172:refnum<class "Text File.lvclass">, "Accessors:Memory Set"=w170:bool, "Accessors:play mode"=w169:u8)  [unwired: 1 in, 2 out]
        n67 = case shown="거짓" w170 {
          tunnel: w172 -> [w179 w243]
          tunnel: [w178 w242] -> w171
          tunnel: [w177 w241] -> w167
          tunnel: [w176 _] -> w166
          tunnel: "Voltage Range" -> [w175 _]
          tunnel: w169 -> [w174 _]
          frame False {
            n68 = case shown="1" w174 {
              tunnel: w179 -> [w200 w232]
              tunnel: [w185 w231] -> w178
              tunnel: [w184 w227] -> w177
              tunnel: [w188 w226] -> w176
              tunnel: w175 -> [w180 w225]
              frame 1 {
                # "PWL"
                n69 = property class="Text File.lvclass"(reference=w200) -> (reference out=w187:refnum<class "Text File.lvclass">, "Accessors:Text_File_PWL"=w192:T1, "Accessors:play mode"=w199:u8, "Accessors:sampling rate"=w190:dbl)  [unwired: 1 in, 1 out]
                n70 = Array Size(array=w192) -> (size(s)=w195:i32)
                n71 = for {
                  tunnel: [w223] -> w197 mode=indexing
                  shift-right: [w211] -> _
                  shift-left: 0.0 ("Amplitude") -> [w212]
                  tunnel: [w222] -> _ mode=concatenating
                  tunnel: w192 -> [w220] mode=indexing
                  tunnel: w180 -> [w213]
                  tunnel: w199 -> [w215]
                  tunnel: w190 -> [w214]
                  n72 = Unbundle By Name(w220) -> ("Shape"=w219:u16, "Ramp"=w218:u16, "Amplitude"=w211:dbl, "Frequency"=w217:dbl, "Cycle"=w216:dbl)
                  n73 = property class="PWL_DW7802.lvclass"(reference=refnum<class "PWL_DW7802.lvclass"> refnum ("PWL_DW7802.lvclass"), "Accessors:waveform type"=w219, "Accessors:repeat type"=w218, "Accessors:scale"=w211, "Accessors:frequency"=w217, "Accessors:cycle"=w216, "Accessors:play mode"=w215, "Accessors:sampling rate"=w214, "Accessors:voltage range"=w213, "Accessors:previous pwl scale"=w212) -> (reference out=w224:refnum<class "PWL_DW7802.lvclass">)  [unwired: 1 in, 1 out]
                  n74 = call-dynamic "get waveform - 8bit.vi"("PWL_DW7802 입력"=w224) -> ("8bit memory data"=w222:u8[], "PWL_DW7802 출력"=w223:refnum<class "PWL_DW7802.lvclass">)  [unwired: 7 in, 2 out]
                }
                n75 = property on="Voltage Range" class="Ring (엄격한)"() -> ("StringsAndValues[]"=w181:T5)  [unwired: 2 in, 2 out]
                n76 = To Long Integer(number=w195) -> (32bit integer=w193:i32)
                n77 = for {
                  N: w193 -> [_]
                  tunnel: [w206] -> w196 mode=indexing
                  i -> [w207]
                  n78 = Increment(x=w207) -> (x+1=w206:i32)
                }
                n79 = for {
                  tunnel: w181 -> [w205] mode=indexing
                  tunnel: w180 -> [w204]
                  tunnel: [w201] -> w182
                  i -> [w201]
                  stop <- w202 stop-if-true
                  n80 = Unbundle By Name(w205) -> ("Value"=w203:dbl)
                  n81 = Equal?(x=w204, y=w203) -> (x = y?=w202:bool)
                }
                n82 = Number To Decimal String(number=w196) -> (decimal integer string=w194:string[])  [unwired: 1 in]
                n83 = property on="WF Seq_PWL Listbox" class="MCListbox (엄격한)"("RowHdrs[]"=w194) -> ()  [unwired: 2 in, 2 out]
                n84 = property on="WF Seq_PWL_DW7802 3" class="Arr (엄격한)"("Value"=w192, "Number of Rows"=w193) -> ()  [unwired: 2 in, 2 out]
                n85 = for {
                  tunnel: w197 -> [w210] mode=indexing
                  tunnel: [w208] -> w191 mode=concatenating
                  n86 = call-dynamic "get waveform - voltage range scaled.vi"("Waveform Obj 입력"=w210) -> ("scaled waveform"=w209:waveform(dbl))  [unwired: 8 in, 2 out]
                  n87 = Unbundle By Name(w209) -> ("Y"=w208:dbl[])
                }
                n88 = Reciprocal(x=w190) -> (1/x=w189:dbl)
                n89 = Bundle By Name("Y"=w191, "dt"=w189) -> (w188:waveform(dbl))  [unwired: 1 in]
                n90 = property class="Text File.lvclass"(reference=w187, "Accessors:voltage idx"=w182, "Accessors:voltage range"=w180) -> (reference out=w183:refnum<class "Text File.lvclass">)  [unwired: 1 in, 1 out]
                n91 = call "Text File_Change the Header.vi"("참조 출력"=w183) -> ("참조 출력 2"=w186:refnum<class "Text File.lvclass">)  [unwired: 9 in, 1 out]
                n92 = property class="Text File.lvclass"(reference=w186) -> (reference out=w185:refnum<class "Text File.lvclass">, "Accessors:Text_Data"=w184:string)  [unwired: 1 in, 1 out]
              }
              frame 0, Default {
                # "기본"
                n93 = property on="Voltage Range" class="Ring (엄격한)"() -> ("StringsAndValues[]"=w234:T5)  [unwired: 2 in, 2 out]
                n94 = for {
                  tunnel: w234 -> [w240] mode=indexing
                  tunnel: w225 -> [w239]
                  tunnel: [w236] -> w233
                  i -> [w236]
                  stop <- w237 stop-if-true
                  n95 = Unbundle By Name(w240) -> ("Value"=w238:dbl)
                  n96 = Equal?(x=w239, y=w238) -> (x = y?=w237:bool)
                }
                n97 = property class="Text File.lvclass"(reference=w232, "Accessors:wait"="Wait", "Accessors:voltage range"=w225, "Accessors:voltage idx"=w233) -> (reference out=w230:refnum<class "Text File.lvclass">)  [unwired: 1 in, 1 out]
                n98 = call "Text File_Change the Header.vi"("참조 출력"=w230) -> ("참조 출력 2"=w229:refnum<class "Text File.lvclass">)  [unwired: 9 in, 1 out]
                n99 = property class="Text File.lvclass"(reference=w229) -> (reference out=w228:refnum<class "Text File.lvclass">, "Accessors:Text_Data"=w227:string)  [unwired: 1 in, 1 out]
                n100 = call-dynamic "get waveform - voltage range scaled.vi"("Text File 입력"=w228) -> ("scaled waveform"=w226:waveform(dbl), "Text File 출력"=w231:refnum<class "Text File.lvclass">)  [unwired: 8 in, 1 out]
              }
            }
          }
          frame True {
            n101 = property class="Text File.lvclass"(reference=w243) -> (reference out=w242:refnum<class "Text File.lvclass">, "Accessors:Text_Data"=w241:string)  [unwired: 1 in, 1 out]
            n102 = property on="Apply" class="Bool"("DisabledEnum"=T3."Disabled and Grayed Out" ("비활성화"), "TipStrip"="Memory Form data cannot be loaded" ("메시지")) -> ()  [unwired: 2 in, 2 out]
          }
        }
        "Graph" <- w166
        n103 = local write "TXT_Preview"(w167) -> ()
      }
    }
    "Apply?" <- w118
    n104 = Or(x=w121, y=w119) -> (x .or. y?=w120:bool)
  }
  "error out" <- w11
  "Text File 출력" <- w23
  n105 = control-ref of="이 VI"() -> (w13:refnum<vi>)
  n106 = property class="VI"(reference=w13, error in=w11, "Front Panel.Title"="Import Manger_TextFile" ("프런트패널 윈도우:제목")) -> ()  [unwired: 2 out]
